vi "Voltage and Current Ring Chooser.vi"(8 "error in (no error)":errorcluster, 11 "Yokogawa WT500 in":refnum<class "Yokogawa WT500.lvclass">) -> (0 "error out":errorcluster, 1 "Current Strings And Values []":T1, 2 "Voltage Strings And Values []":T1, 3 "Yokogawa WT500 out":refnum<class "Yokogawa WT500.lvclass">)   [LabVIEW 2013, in "Universal Power Meter.lvlib" / "Yokogawa WT500.lvlib" / "Yokogawa WT500.lvclass"]
uses:
  Yokogawa WT500.lvclass
  <vilib>/Utility/miscctls.llb/LVStringsAndValuesArrayTypeDef_U16.ctl
panel:
  in  "Voltage Range (8: 1000V)":u16(ring)=8 items=["AUTO", "15", "30", "60", "100", "150", "300", "600", "1000"]
  in  "Current Range (7: 40A)":u16(ring)=7 items=["AUTO", "500 mA", "1 A", "2 A", "5 A", "10 A", "20 A", "40 A"]
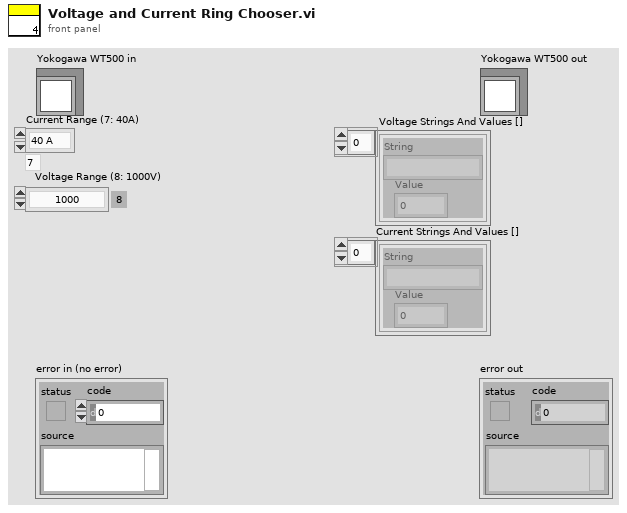
[diagram p1: front panel]
types:
  T1 = typedef "LVStringsAndValuesArrayTypeDef_U16.ctl" = cluster{"String":string, "Value":u16}[]
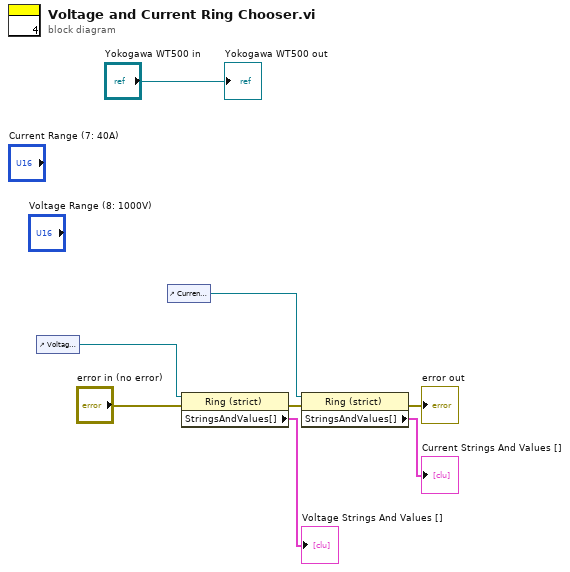
[diagram p0: block diagram]
diagram:
  n1 = control-ref of="Voltage Range (8: 1000V)"() -> (w7:refnum<vi>)
  n2 = control-ref of="Current Range (7: 40A)"() -> (w3:refnum<vi>)
  n3 = property class="Ring (strict)"(reference=w7, error in="error in (no error)") -> (error out=w4:errorcluster, "StringsAndValues[]"=→"Voltage Strings And Values []":T1)  [unwired: 1 out]
  n4 = property class="Ring (strict)"(reference=w3, error in=w4) -> (error out=→"error out":errorcluster, "StringsAndValues[]"=→"Current Strings And Values []":T1)  [unwired: 1 out]
  "Yokogawa WT500 out" <- "Yokogawa WT500 in"
